vi "初始化水样搜索起始时间.vi"(8 "error in (no error)":errorcluster caption="错误输入（无错误）", 11 "参数数值":T3={"CODMn"=TRUE, "CODCr"=TRUE, "DO"=TRUE, "铜"=TRUE, "PH"=TRUE, "氨氮"=TRUE, "比电导率"=TRUE, "水温"=TRUE, "盐度(海水)"=TRUE, "浊度"=TRUE, "总氮"=TRUE, "总磷"=TRUE, "叶绿素a"=TRUE, "藻密度"=TRUE, "水位"=TRUE, "流速"=TRUE, "瞬时流量"=TRUE, "累积流量"=TRUE}) -> (0 "error out":errorcluster caption="错误输出", 3 "数值":i32)   [LabVIEW 2016, in "数据传输系统.lvlib"]
uses:
  <vilib>/Utility/config.llb/Read Key (String).vi
  <vilib>/Utility/config.llb/NI_LVConfig.lvlib
panel:
  in  "重发时间":T1(ring)
  in  "重发日期":T2(ring)
  in  "每周自动重发":bool=TRUE
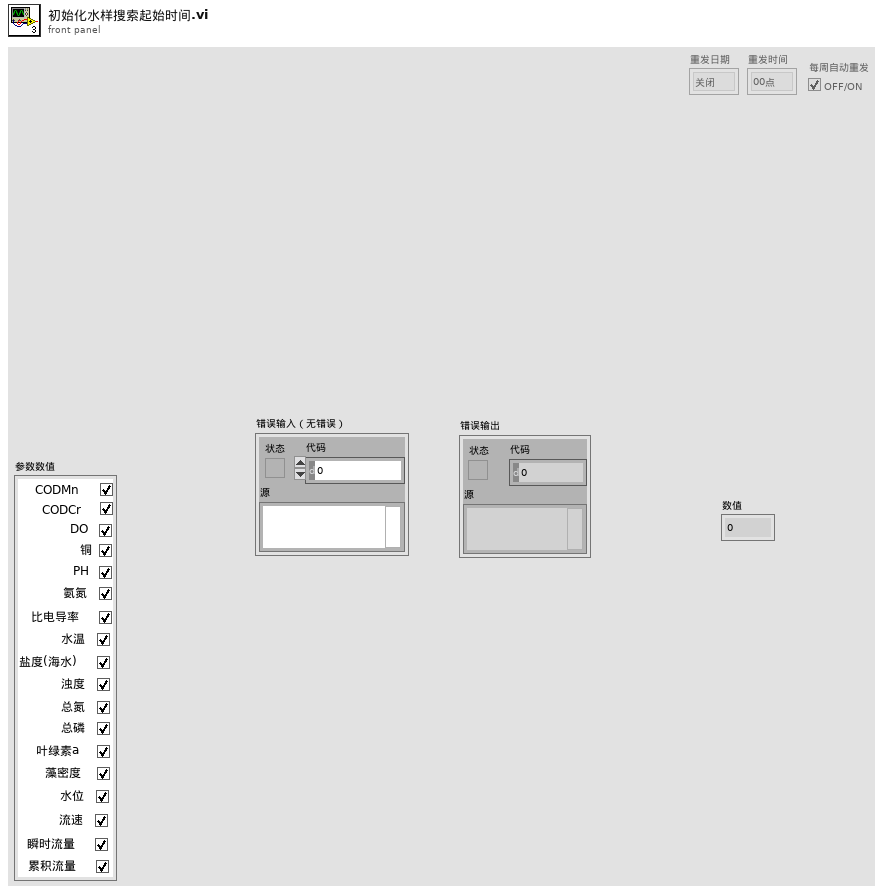
[diagram p1: front panel]
types:
  T1 = enum16{"00点", "01点", "02点", "03点", "04点", "05点", "06点", "07点", "08点", "09点", "10点", "11点", "12点", "13点", "14点", "15点", "16点", "17点", "18点", "19点", "20点", "21点", "22点", "23点"}
  T2 = enum16{"关闭", "星期日", "星期一", "星期二", "星期三", "星期四", "星期五", "星期六"}
  T3 = cluster{"CODMn":bool, "CODCr":bool, "DO":bool, "铜":bool, "PH":bool, "氨氮":bool, "比电导率":bool, "水温":bool, "盐度(海水)":bool, "浊度":bool, "总氮":bool, "总磷":bool, "叶绿素a":bool, "藻密度":bool, "水位":bool, "流速":bool, "瞬时流量":bool, "累积流量":bool}
  T4 = typedef "NI_LVConfig.lvlib/Config Data RefNum.ctl" = refnum<k1>
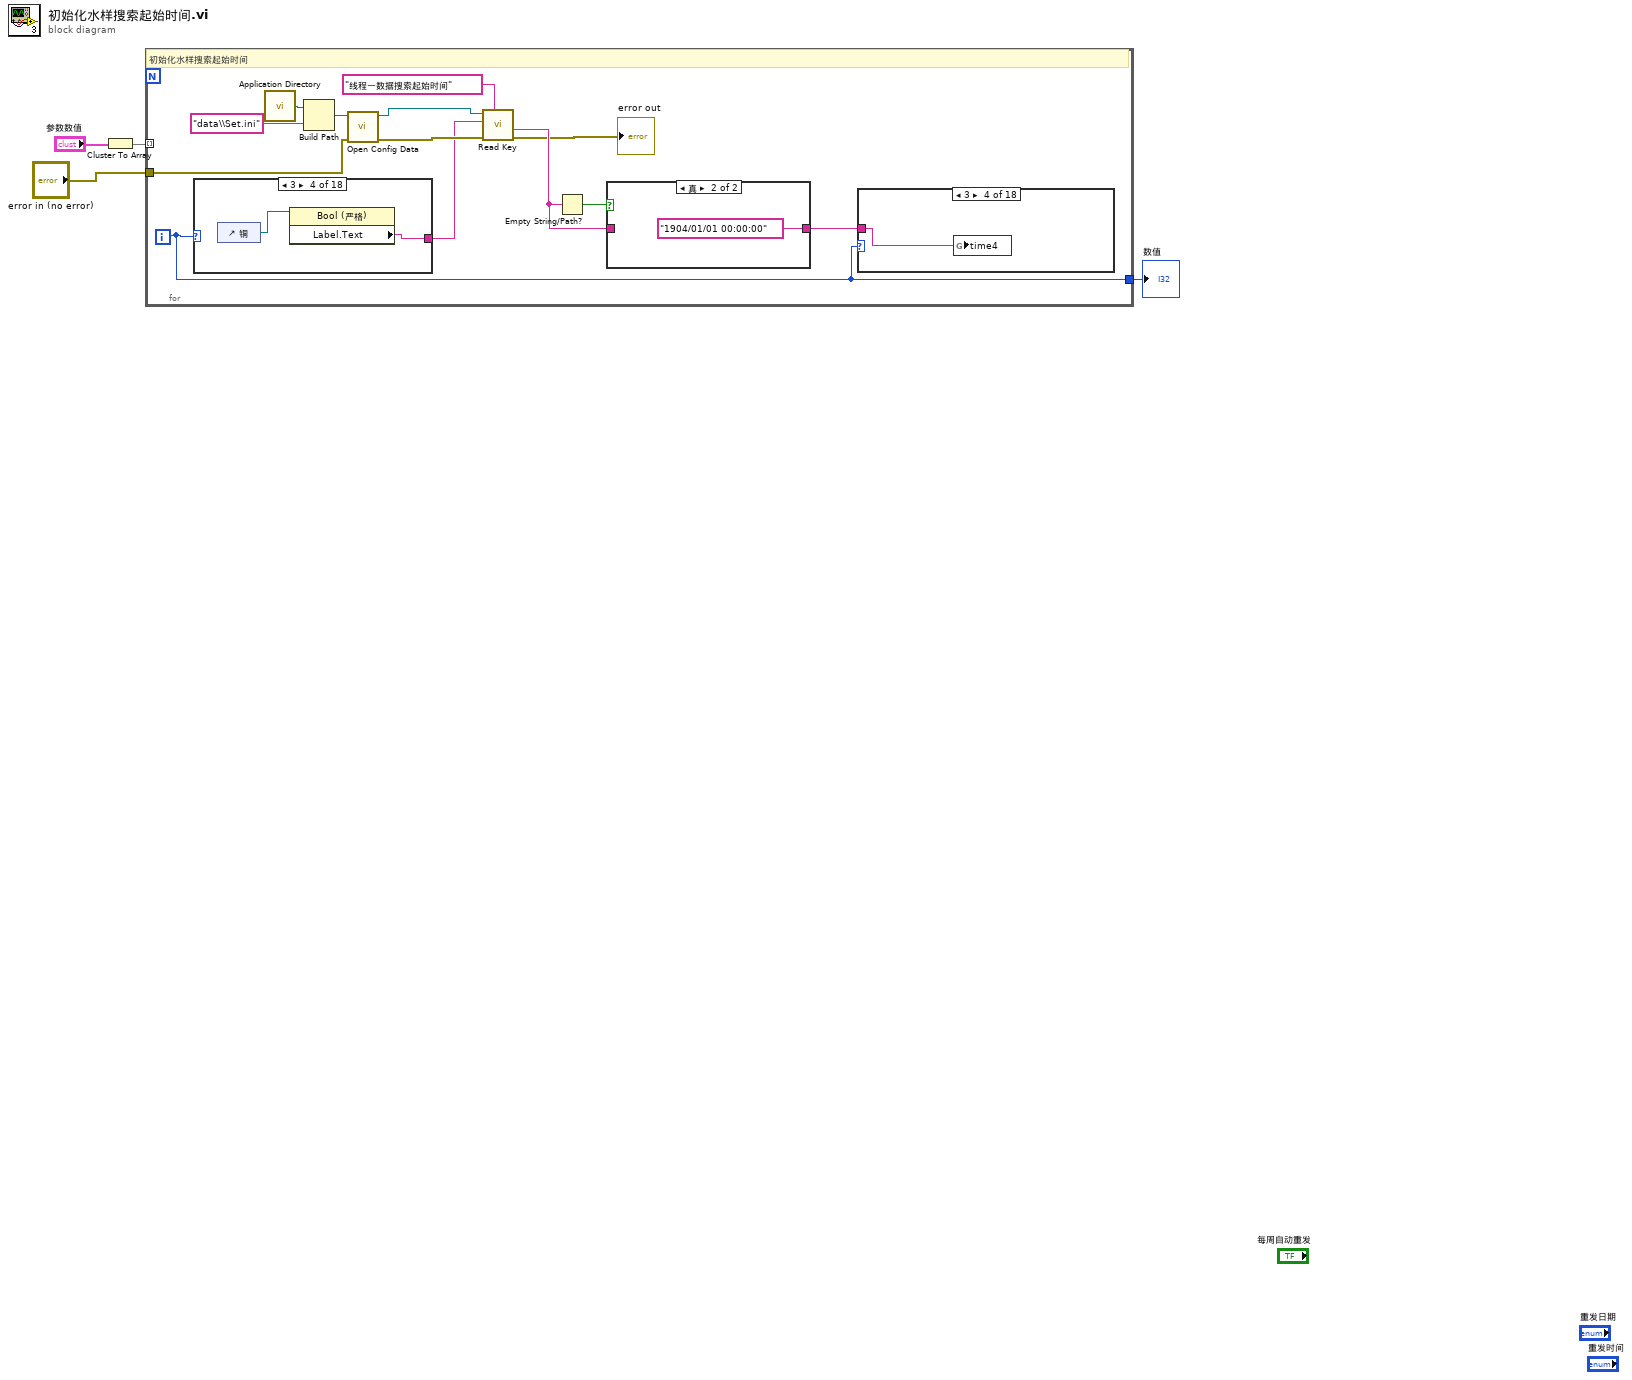
[diagram p0: block diagram]
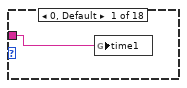
[diagram p3: hidden frame]
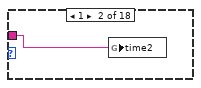
[diagram p4: hidden frame]
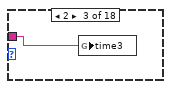
[diagram p5: hidden frame]
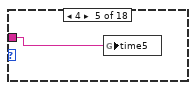
[diagram p6: hidden frame]
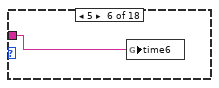
[diagram p7: hidden frame]
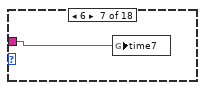
[diagram p8: hidden frame]
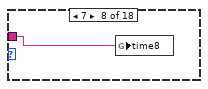
[diagram p9: hidden frame]
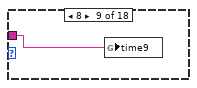
[diagram p10: hidden frame]
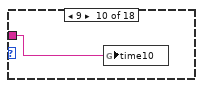
[diagram p11: hidden frame]
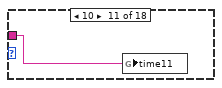
[diagram p12: hidden frame]
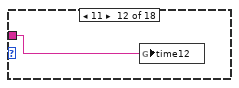
[diagram p13: hidden frame]
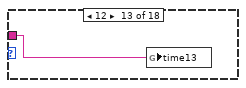
[diagram p14: hidden frame]
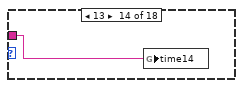
[diagram p15: hidden frame]
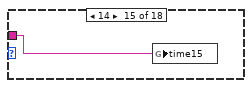
[diagram p16: hidden frame]
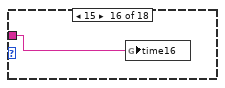
[diagram p17: hidden frame]
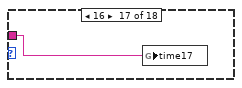
[diagram p18: hidden frame]
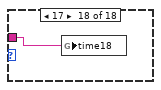
[diagram p19: hidden frame]
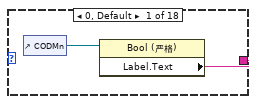
[diagram p20: hidden frame]
diagram:
  n1 = Cluster To Array(cluster="参数数值") -> (array=w3:bool[])
  n2 = for {
    tunnel: w3 -> [_] mode=indexing
    tunnel: [w7] -> w2
    tunnel: "error in (no error)" -> [w6]
    i -> [w7]
    # "初始化水样搜索起始时间"
    n3 = case shown="3" w7 {
      tunnel: [w38 w40 w42 w44 w46 w48 w50 w52 w54 w56 w58 w60 w62 w64 w66 w68 w70 w72] -> w11
      frame 0, Default {
        n4 = control-ref of="CODMn"() -> (w39:refnum<vi>)
        n5 = property class="Bool (严格)"(reference=w39) -> ("Label.Text"=w38:string)  [unwired: 1 in, 2 out]
      }
      frame 1 {
        n6 = control-ref of="CODCr"() -> (w41:refnum<vi>)
        n7 = property class="Bool (严格)"(reference=w41) -> ("Label.Text"=w40:string)  [unwired: 1 in, 2 out]
      }
      frame 2 {
        n8 = control-ref of="DO"() -> (w43:refnum<vi>)
        n9 = property class="Bool (严格)"(reference=w43) -> ("Label.Text"=w42:string)  [unwired: 1 in, 2 out]
      }
      frame 3 {
        n10 = control-ref of="铜"() -> (w45:refnum<vi>)
        n11 = property class="Bool (严格)"(reference=w45) -> ("Label.Text"=w44:string)  [unwired: 1 in, 2 out]
      }
      frame 4 {
        n12 = control-ref of="PH"() -> (w47:refnum<vi>)
        n13 = property class="Bool (严格)"(reference=w47) -> ("Label.Text"=w46:string)  [unwired: 1 in, 2 out]
      }
      frame 5 {
        n14 = control-ref of="氨氮"() -> (w49:refnum<vi>)
        n15 = property class="Bool (严格)"(reference=w49) -> ("Label.Text"=w48:string)  [unwired: 1 in, 2 out]
      }
      frame 6 {
        n16 = control-ref of="比电导率"() -> (w51:refnum<vi>)
        n17 = property class="Bool (严格)"(reference=w51) -> ("Label.Text"=w50:string)  [unwired: 1 in, 2 out]
      }
      frame 7 {
        n18 = control-ref of="水温"() -> (w53:refnum<vi>)
        n19 = property class="Bool (严格)"(reference=w53) -> ("Label.Text"=w52:string)  [unwired: 1 in, 2 out]
      }
      frame 8 {
        n20 = control-ref of="盐度(海水)"() -> (w55:refnum<vi>)
        n21 = property class="Bool (严格)"(reference=w55) -> ("Label.Text"=w54:string)  [unwired: 1 in, 2 out]
      }
      frame 9 {
        n22 = control-ref of="浊度"() -> (w57:refnum<vi>)
        n23 = property class="Bool (严格)"(reference=w57) -> ("Label.Text"=w56:string)  [unwired: 1 in, 2 out]
      }
      frame 10 {
        n24 = control-ref of="总氮"() -> (w59:refnum<vi>)
        n25 = property class="Bool (严格)"(reference=w59) -> ("Label.Text"=w58:string)  [unwired: 1 in, 2 out]
      }
      frame 11 {
        n26 = control-ref of="总磷"() -> (w61:refnum<vi>)
        n27 = property class="Bool (严格)"(reference=w61) -> ("Label.Text"=w60:string)  [unwired: 1 in, 2 out]
      }
      frame 12 {
        n28 = control-ref of="叶绿素a"() -> (w63:refnum<vi>)
        n29 = property class="Bool (严格)"(reference=w63) -> ("Label.Text"=w62:string)  [unwired: 1 in, 2 out]
      }
      frame 13 {
        n30 = control-ref of="藻密度"() -> (w65:refnum<vi>)
        n31 = property class="Bool (严格)"(reference=w65) -> ("Label.Text"=w64:string)  [unwired: 1 in, 2 out]
      }
      frame 14 {
        n32 = control-ref of="水位"() -> (w67:refnum<vi>)
        n33 = property class="Bool (严格)"(reference=w67) -> ("Label.Text"=w66:string)  [unwired: 1 in, 2 out]
      }
      frame 15 {
        n34 = control-ref of="流速"() -> (w69:refnum<vi>)
        n35 = property class="Bool (严格)"(reference=w69) -> ("Label.Text"=w68:string)  [unwired: 1 in, 2 out]
      }
      frame 16 {
        n36 = control-ref of="瞬时流量"() -> (w71:refnum<vi>)
        n37 = property class="Bool (严格)"(reference=w71) -> ("Label.Text"=w70:string)  [unwired: 1 in, 2 out]
      }
      frame 17 {
        n38 = control-ref of="累积流量"() -> (w73:refnum<vi>)
        n39 = property class="Bool (严格)"(reference=w73) -> ("Label.Text"=w72:string)  [unwired: 1 in, 2 out]
      }
    }
    n40 = call <vilib>:"Application Directory.vi"() -> ("Application Directory"=w17:path)
    n41 = Build Path(base path=w17, name or relative path="data\\Set.ini" ("名称或相对路径")) -> (appended path=w15:path)
    n42 = call <vilib>:"Open Config Data.vi"("error in (no error)"=w6, "configuration file path"=w15) -> ("error out"=w13:errorcluster, "refnum"=w14:T4)  [unwired: 7 in, 1 out]
    n43 = call-poly <vilib>:"Read Key.vi"("section"="线程一数据搜索起始时间", "error in (no error)"=w13, "key"=w11, "refnum"=w14) -> ("error out"=→"error out":errorcluster, "value"=w8:string)  [unwired: 4 in, 2 out]
    n44 = Empty String/Path?(string/path=w8) -> (empty?=w10:bool)
    n45 = case shown="真" w10 {
      tunnel: [w18 "1904/01/01 00:00:00"] -> w9
      tunnel: w8 -> [w18 _]
      frame False {
      }
      frame True {
      }
    }
    n46 = case shown="3" w7 {
      tunnel: w9 -> [w20 w21 w22 w23 w24 w25 w26 w27 w28 w29 w30 w31 w32 w33 w34 w35 w36 w37]
      frame 0, Default {
        n47 = global write "全局 水样时间.vi" "time1"(w20) -> ()
      }
      frame 1 {
        n48 = global write "全局 水样时间.vi" "time2"(w21) -> ()
      }
      frame 2 {
        n49 = global write "全局 水样时间.vi" "time3"(w22) -> ()
      }
      frame 3 {
        n50 = global write "全局 水样时间.vi" "time4"(w23) -> ()
      }
      frame 4 {
        n51 = global write "全局 水样时间.vi" "time5"(w24) -> ()
      }
      frame 5 {
        n52 = global write "全局 水样时间.vi" "time6"(w25) -> ()
      }
      frame 6 {
        n53 = global write "全局 水样时间.vi" "time7"(w26) -> ()
      }
      frame 7 {
        n54 = global write "全局 水样时间.vi" "time8"(w27) -> ()
      }
      frame 8 {
        n55 = global write "全局 水样时间.vi" "time9"(w28) -> ()
      }
      frame 9 {
        n56 = global write "全局 水样时间.vi" "time10"(w29) -> ()
      }
      frame 10 {
        n57 = global write "全局 水样时间.vi" "time11"(w30) -> ()
      }
      frame 11 {
        n58 = global write "全局 水样时间.vi" "time12"(w31) -> ()
      }
      frame 12 {
        n59 = global write "全局 水样时间.vi" "time13"(w32) -> ()
      }
      frame 13 {
        n60 = global write "全局 水样时间.vi" "time14"(w33) -> ()
      }
      frame 14 {
        n61 = global write "全局 水样时间.vi" "time15"(w34) -> ()
      }
      frame 15 {
        n62 = global write "全局 水样时间.vi" "time16"(w35) -> ()
      }
      frame 16 {
        n63 = global write "全局 水样时间.vi" "time17"(w36) -> ()
      }
      frame 17 {
        n64 = global write "全局 水样时间.vi" "time18"(w37) -> ()
      }
    }
  }
  "数值" <- w2
